vi "Blink 2.vi"(8 "Error In":errorcluster, 11 "String control":string="This is text in cotnrol on front panel") -> (0 "Error Out":errorcluster)   [LabVIEW 2014]
panel:
  out "signal out 2":waveform(dbl)
  out "Numeric":i32
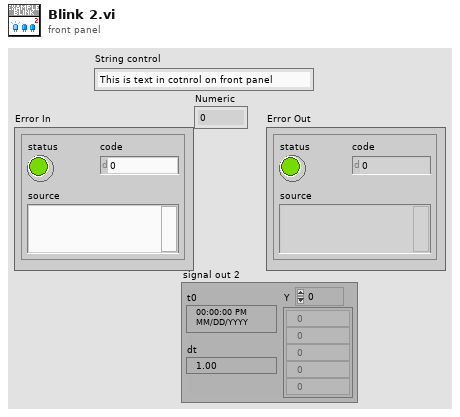
[diagram p1: front panel]
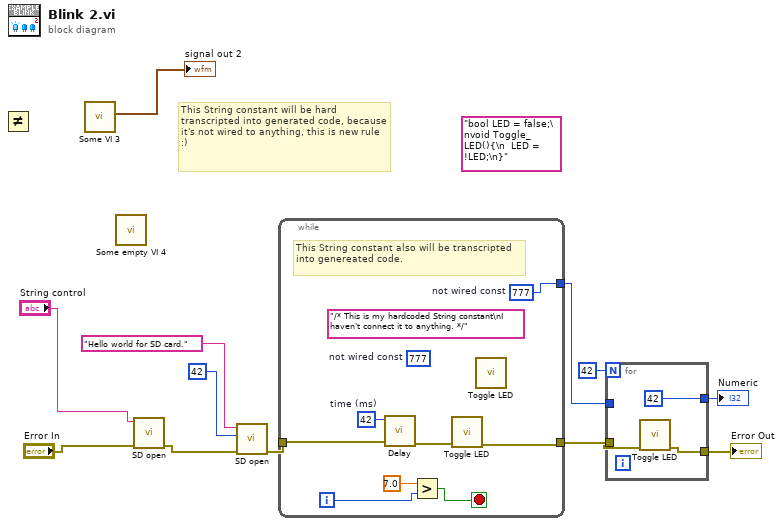
[diagram p0: block diagram]
diagram:
  (unwired) "bool LED = false;\nvoid Toggle_LED(){\n  LED = !LED;\n}"
  # "This String constant will be hard transcripted into generated code, because it's not wired to anything, this is new rule :)"
  n1 = Not Equal?() -> ()  [unwired: 2 in, 1 out]
  n2 = call "Some VI 3.vi"() -> ("signal out 2"=→"signal out 2":waveform(dbl))  [unwired: 10 in, 1 out]
  n3 = call "Some empty VI 4.vi"() -> ()  [unwired: 11 in, 1 out]
  n4 = call "SD open.vi"("Error In"="Error In", "SD card name"="String control") -> ("Error Out"=w8:errorcluster)  [unwired: 9 in]
  n5 = call "SD open.vi"("Error In"=w8, "device address"=42, "SD card name"="Hello world for SD card.") -> ("Error Out"=w12:errorcluster)  [unwired: 8 in]
  n6 = while {
    tunnel: w12 -> [w20]
    tunnel: [w14] -> w6
    tunnel: [w13] -> w3
    i -> [w17]
    stop <- w18 stop-if-true
    w13 = 777  # not wired const
    (unwired) "/* This is my hardcoded String constant\nI haven't connect it to anything. */"
    (unwired) 777  # not wired const
    w15 = 42  # time (ms)
    # "This String constant also will be transcripted into genereated code."
    n7 = call "Delay.vi"("Error In"=w20, "time (ms)"=w15) -> ("Error Out"=w19:errorcluster)  [unwired: 9 in]
    n8 = Greater?(x=7.0, y=w17) -> (0:w18:bool)
    n9 = call "Toggle LED.vi"("Error In"=w19) -> ("Error Out"=w14:errorcluster)  [unwired: 10 in]
    n10 = call "Toggle LED.vi"() -> ()  [unwired: 11 in, 1 out]
  }
  n11 = for {
    N: 42 -> [_]
    tunnel: w6 -> [w23]
    tunnel: [w22] -> w5
    tunnel: w3 -> [_]
    tunnel: [42] -> w2
    n12 = call "Toggle LED.vi"("Error In"=w23) -> ("Error Out"=w22:errorcluster)  [unwired: 10 in]
  }
  "Error Out" <- w5
  "Numeric" <- w2
